vi "Set Thread Interfaces.vi"(10 "Plugin Interfaces":refnum<class "Plugin Interface.lvclass">[](array[class]), 11 "Plugin in":refnum<class "Plugin.lvclass">) -> (3 "Plugin out":refnum<class "Plugin.lvclass">)   [LabVIEW 2020, in "DSF Core.lvlib" / "Plugin.lvclass"]
uses:
  Plugin.lvclass
  Interface/Plugin/Plugin Interface.lvclass
  Plugin.lvclass/Plugin.ctl
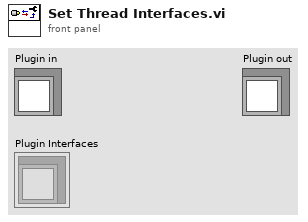
[diagram p1: front panel]
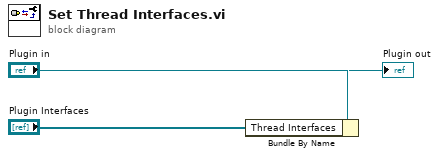
[diagram p0: block diagram]
diagram:
  n1 = Bundle By Name(cluster="Plugin in", "Thread Interfaces"="Plugin Interfaces") -> (→"Plugin out":refnum<class "Plugin.lvclass">)
